vi "BoxBegin.vi"   [LabVIEW 2023]
uses:
  <vilib>/Rock Robotics/WPI/ThirdParty/REV Robotics/REVLib/Typedef/Spark MAX Sensor Type.ctl
  <vilib>/Rock Robotics/WPI/ThirdParty/REV Robotics/REVLib/Typedef/Spark MAX Limit Direction.ctl
  <vilib>/Rock Robotics/WPI/ThirdParty/REV Robotics/REVLib/Typedef/Spark MAX Idle Mode.ctl
  <vilib>/Rock Robotics/WPI/ThirdParty/REV Robotics/REVLib/Typedef/Spark MAX Limit Switch Polarity.ctl
  <vilib>/Rock Robotics/WPI/ThirdParty/REV Robotics/REVLib/Typedef/Spark MAX Motor Type.ctl
types:
  T1 = typedef "Spark MAX Sensor Type.ctl" = enum16{"No Sensor", "Hall Sensor", "Encoder", "-Not Available-", "Analog", "Alternate Encoder", "Duty Cycle"}
  T2 = typedef "Spark MAX Limit Direction.ctl" = enum16{"Forward Limit", "Reverse Limit"}
  T3 = typedef "Spark MAX Limit Switch Polarity.ctl" = enum16{"Normally Open", "Normally Closed"}
  T4 = typedef "Spark MAX Idle Mode.ctl" = enum16{"Coast", "Brake"}
  T5 = typedef "Spark MAX Motor Type.ctl" = enum16{"Brushed", "Brushless"}
  T6 = typedef "WPI_MotorControlDeviceRef.ctl" = cluster{"DeviceStatus":errorcluster, "Type":T7, "PWM":cluster{"PWM Channel":T8, "DeadBand":T9}, "CAN":cluster{"Device Number":u8, "SetOutput VI Ref":variant, "GetOutput VI Ref":variant, "Enable VI Ref":variant, "Disable VI Ref":variant, "Data":variant}, "Invert":bool, "DIO PWM":cluster{"PWM \"Enable\" Channel":T8, "DIOChannel":T10, "PWM Rate":dbl}}
  T7 = typedef "WPI_MotorControlType.ctl" = enum16{"PWM", "CAN", "DIO PWM"}
  T8 = typedef "FPGA_DIOPWMChannel.ctl" = enum8{"PWM 0", "PWM 1", "PWM 2", "PWM 3", "PWM 4", "PWM 5", "PWM 6", "PWM 7", "PWM 8", "PWM 9", "PWM MXP 0", "PWM MXP 1", "PWM MXP 2", "PWM MXP 3", "PWM MXP 4", "PWM MXP 5", "PWM MXP 6", "PWM MXP 7", "PWM MXP 8", "PWM MXP 9", "Invalid"}
  T9 = typedef "WPI_PWMDeadband.ctl" = cluster{"Name":string, "maxPositivePwm":i32, "minPositivePwm":i32, "centerPwm":i32, "maxNegativePwm":i32, "minNegativePwm":i32, "angularRange":u16}
  T10 = typedef "FPGA_DIOChannel.ctl" = enum8{"DIO 0", "DIO 1", "DIO 2", "DIO 3", "DIO 4", "DIO 5", "DIO 6", "DIO 7", "DIO 8", "DIO 9", "DIO MXP 0", "DIO MXP 1", "DIO MXP 2", "DIO MXP 3", "DIO MXP 4", "DIO MXP 5", "DIO MXP 6", "DIO MXP 7", "DIO MXP 8", "DIO MXP 9", "DIO MXP 10", "DIO MXP 11", "DIO MXP 12", "DIO MXP 13", "DIO MXP 14", "DIO MXP 15", "SPI Port CS1", "SPI Port CS2", "SPI Port CS3", "SPI Port MISO", "SPI Port MOSI", "Invalid"}
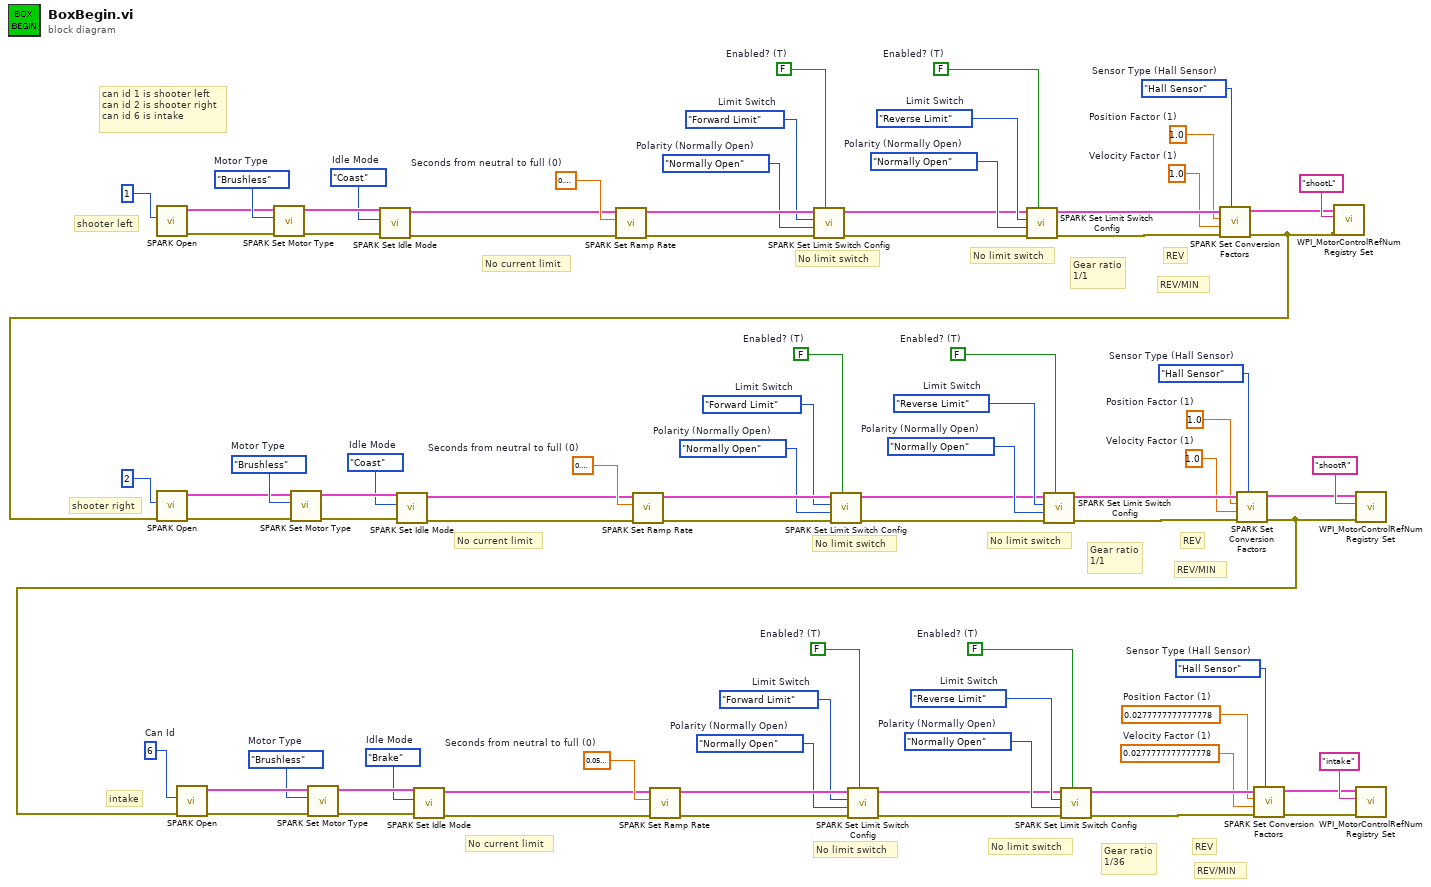
[diagram p0: block diagram]
diagram:
  w8 = 1.0  # Position Factor (1)
  w9 = 1.0  # Velocity Factor (1)
  w10 = Spark_MAX_Sensor_Type."Hall Sensor"  # Sensor Type (Hall Sensor)
  w15 = Spark_MAX_Limit_Direction."Reverse Limit"  # Limit Switch
  w16 = Spark_MAX_Limit_Switch_Polarity."Normally Open"  # Polarity (Normally Open)
  w17 = FALSE  # Enabled? (T)
  w18 = Spark_MAX_Limit_Direction."Forward Limit"  # Limit Switch
  w19 = Spark_MAX_Limit_Switch_Polarity."Normally Open"  # Polarity (Normally Open)
  w20 = FALSE  # Enabled? (T)
  w23 = sgl 0.1  # Seconds from neutral to full (0)
  w24 = Spark_MAX_Idle_Mode."Coast"  # Idle Mode
  w25 = Spark_MAX_Motor_Type."Brushless"  # Motor Type
  w33 = 1.0  # Position Factor (1)
  w34 = 1.0  # Velocity Factor (1)
  w35 = Spark_MAX_Sensor_Type."Hall Sensor"  # Sensor Type (Hall Sensor)
  w40 = Spark_MAX_Limit_Direction."Reverse Limit"  # Limit Switch
  w41 = Spark_MAX_Limit_Switch_Polarity."Normally Open"  # Polarity (Normally Open)
  w42 = FALSE  # Enabled? (T)
  w43 = Spark_MAX_Limit_Direction."Forward Limit"  # Limit Switch
  w44 = Spark_MAX_Limit_Switch_Polarity."Normally Open"  # Polarity (Normally Open)
  w45 = FALSE  # Enabled? (T)
  w48 = sgl 0.1  # Seconds from neutral to full (0)
  w49 = Spark_MAX_Idle_Mode."Coast"  # Idle Mode
  w50 = Spark_MAX_Motor_Type."Brushless"  # Motor Type
  w57 = 0.0277777777777778  # Position Factor (1)
  w58 = 0.0277777777777778  # Velocity Factor (1)
  w59 = Spark_MAX_Sensor_Type."Hall Sensor"  # Sensor Type (Hall Sensor)
  w64 = Spark_MAX_Limit_Direction."Reverse Limit"  # Limit Switch
  w65 = Spark_MAX_Limit_Switch_Polarity."Normally Open"  # Polarity (Normally Open)
  w66 = FALSE  # Enabled? (T)
  w67 = Spark_MAX_Limit_Direction."Forward Limit"  # Limit Switch
  w68 = Spark_MAX_Limit_Switch_Polarity."Normally Open"  # Polarity (Normally Open)
  w69 = FALSE  # Enabled? (T)
  w72 = sgl 0.06  # Seconds from neutral to full (0)
  w74 = Spark_MAX_Idle_Mode."Brake"  # Idle Mode
  w75 = Spark_MAX_Motor_Type."Brushless"  # Motor Type
  w81 = 6  # Can Id
  # "No current limit"
  # "No current limit"
  # "No current limit"
  # "No limit switch"
  # "No limit switch"
  # "Gear ratio\n1/1"
  # "REV/MIN"
  # "REV"
  # "No limit switch"
  # "No limit switch"
  # "No limit switch"
  # "No limit switch"
  # "Gear ratio\n1/1"
  # "REV/MIN"
  # "REV"
  # "Gear ratio\n1/36"
  # "REV/MIN"
  # "REV"
  # "intake"
  # "shooter right"
  # "shooter left"
  # "can id 1 is shooter left\ncan id 2 is shooter right\ncan id 6 is intake"
  n1 = call <vilib>:"SPARK Open.vi"("Device Number"=1) -> ("error out"=w4:errorcluster, "MotorControlDeviceRef"=w5:T6)  [unwired: 9 in]
  n2 = call <vilib>:"SPARK Set Motor Type.vi"("error in (no error)"=w4, "Motor Type"=w25, "MotorControlDevRef"=w5) -> ("error out"=w26:errorcluster, "MotorControlDeviceRef"=w27:T6)  [unwired: 7 in]
  n3 = call <vilib>:"SPARK Set Idle Mode.vi"("error in (no error)"=w26, "Idle Mode"=w24, "MotorControlDeviceRef in"=w27) -> ("error out"=w6:errorcluster, "MotorControlDeviceRef out"=w7:T6)  [unwired: 7 in]
  n4 = call <vilib>:"SPARK Set Ramp Rate.vi"("error in (no error)"=w6, "Seconds from neutral to full (0)"=w23, "MotorControlDeviceRef in"=w7) -> ("error out"=w21:errorcluster, "MotorControlDeviceRef"=w22:T6)  [unwired: 7 in]
  n5 = call <vilib>:"SPARK Set Limit Switch Config.vi"("Enabled? (T)"=w20, "error in (no error)"=w21, "Polarity (Normally Open)"=w19, "Limit Switch"=w18, "MotorControlDeviceRef in"=w22) -> ("error out"=w13:errorcluster, "MotorControlDeviceRef out"=w14:T6)  [unwired: 5 in]
  n6 = call <vilib>:"SPARK Set Limit Switch Config.vi"("Enabled? (T)"=w17, "error in (no error)"=w13, "Polarity (Normally Open)"=w16, "Limit Switch"=w15, "MotorControlDeviceRef in"=w14) -> ("error out"=w11:errorcluster, "MotorControlDeviceRef out"=w12:T6)  [unwired: 5 in]
  n7 = call <vilib>:"SPARK Set Conversion Factors.vi"("Sensor Type (Hall Sensor)"=w10, "error in (no error)"=w11, "Velocity Factor (1)"=w9, "Position Factor (1)"=w8, "MotorControlDeviceRef in"=w12) -> ("error out"=w1:errorcluster, "MotorControlDeviceRef out"=w3:T6)  [unwired: 5 in]
  n8 = call <vilib>:"SPARK Open.vi"("error in (no error)"=w1, "Device Number"=2) -> ("error out"=w29:errorcluster, "MotorControlDeviceRef"=w30:T6)  [unwired: 8 in]
  n9 = call <vilib>:"SPARK Set Motor Type.vi"("error in (no error)"=w29, "Motor Type"=w50, "MotorControlDevRef"=w30) -> ("error out"=w51:errorcluster, "MotorControlDeviceRef"=w52:T6)  [unwired: 7 in]
  n10 = call <vilib>:"SPARK Set Idle Mode.vi"("error in (no error)"=w51, "Idle Mode"=w49, "MotorControlDeviceRef in"=w52) -> ("error out"=w31:errorcluster, "MotorControlDeviceRef out"=w32:T6)  [unwired: 7 in]
  n11 = call <vilib>:"SPARK Set Ramp Rate.vi"("error in (no error)"=w31, "Seconds from neutral to full (0)"=w48, "MotorControlDeviceRef in"=w32) -> ("error out"=w46:errorcluster, "MotorControlDeviceRef"=w47:T6)  [unwired: 7 in]
  n12 = call <vilib>:"SPARK Set Limit Switch Config.vi"("Enabled? (T)"=w45, "error in (no error)"=w46, "Polarity (Normally Open)"=w44, "Limit Switch"=w43, "MotorControlDeviceRef in"=w47) -> ("error out"=w38:errorcluster, "MotorControlDeviceRef out"=w39:T6)  [unwired: 5 in]
  n13 = call <vilib>:"SPARK Set Limit Switch Config.vi"("Enabled? (T)"=w42, "error in (no error)"=w38, "Polarity (Normally Open)"=w41, "Limit Switch"=w40, "MotorControlDeviceRef in"=w39) -> ("error out"=w36:errorcluster, "MotorControlDeviceRef out"=w37:T6)  [unwired: 5 in]
  n14 = call <vilib>:"SPARK Set Conversion Factors.vi"("Sensor Type (Hall Sensor)"=w35, "error in (no error)"=w36, "Velocity Factor (1)"=w34, "Position Factor (1)"=w33, "MotorControlDeviceRef in"=w37) -> ("error out"=w2:errorcluster, "MotorControlDeviceRef out"=w28:T6)  [unwired: 5 in]
  n15 = call <vilib>:"SPARK Open.vi"("error in (no error)"=w2, "Device Number"=w81) -> ("error out"=w77:errorcluster, "MotorControlDeviceRef"=w79:T6)  [unwired: 8 in]
  n16 = call <vilib>:"SPARK Set Motor Type.vi"("error in (no error)"=w77, "Motor Type"=w75, "MotorControlDevRef"=w79) -> ("error out"=w76:errorcluster, "MotorControlDeviceRef"=w78:T6)  [unwired: 7 in]
  n17 = call <vilib>:"SPARK Set Idle Mode.vi"("error in (no error)"=w76, "Idle Mode"=w74, "MotorControlDeviceRef in"=w78) -> ("error out"=w53:errorcluster, "MotorControlDeviceRef out"=w54:T6)  [unwired: 7 in]
  n18 = call <vilib>:"SPARK Set Ramp Rate.vi"("error in (no error)"=w53, "Seconds from neutral to full (0)"=w72, "MotorControlDeviceRef in"=w54) -> ("error out"=w70:errorcluster, "MotorControlDeviceRef"=w71:T6)  [unwired: 7 in]
  n19 = call <vilib>:"SPARK Set Limit Switch Config.vi"("Enabled? (T)"=w69, "error in (no error)"=w70, "Polarity (Normally Open)"=w68, "Limit Switch"=w67, "MotorControlDeviceRef in"=w71) -> ("error out"=w62:errorcluster, "MotorControlDeviceRef out"=w63:T6)  [unwired: 5 in]
  n20 = call <vilib>:"SPARK Set Limit Switch Config.vi"("Enabled? (T)"=w66, "error in (no error)"=w62, "Polarity (Normally Open)"=w65, "Limit Switch"=w64, "MotorControlDeviceRef in"=w63) -> ("error out"=w60:errorcluster, "MotorControlDeviceRef out"=w61:T6)  [unwired: 5 in]
  n21 = call <vilib>:"SPARK Set Conversion Factors.vi"("Sensor Type (Hall Sensor)"=w59, "error in (no error)"=w60, "Velocity Factor (1)"=w58, "Position Factor (1)"=w57, "MotorControlDeviceRef in"=w61) -> ("error out"=w55:errorcluster, "MotorControlDeviceRef out"=w56:T6)  [unwired: 5 in]
  n22 = call <vilib>:"WPI_MotorControlRefNum Registry Set.vi"("error in (no error)"=w1, "refnum name"="shootL", "MotorControlDevRef"=w3) -> ()  [unwired: 7 in, 2 out]
  n23 = call <vilib>:"WPI_MotorControlRefNum Registry Set.vi"("error in (no error)"=w2, "refnum name"="shootR", "MotorControlDevRef"=w28) -> ()  [unwired: 7 in, 2 out]
  n24 = call <vilib>:"WPI_MotorControlRefNum Registry Set.vi"("error in (no error)"=w55, "refnum name"="intake", "MotorControlDevRef"=w56) -> ()  [unwired: 7 in, 2 out]
